vi "FFT x(t) to dB,Degrees (1D).vi"(8 "Fs (Hz)":dbl=1.0, 11 "X":dbl[](array[numeric]) format="%.2f") -> (0 "Freq (Hz)":dbl[](array[numeric]), 2 "+Freq Phase of FFT (degrees)":dbl[](array[numeric]) format="%.2f", 3 "+Freq. Mag of FFT (dB rms)":dbl[](array[numeric]) format="%.2f")   [LabVIEW 2020]
uses:
  <vilib>/Analysis/2dsp.llb/Real FFT.vi
  fea094be-e35f-4e8d-ad5d-9d99f41f383c.vi
  LinSpace (x0-dx-npts).vi
  <vilib>/Analysis/NI_AALPro.lvlib
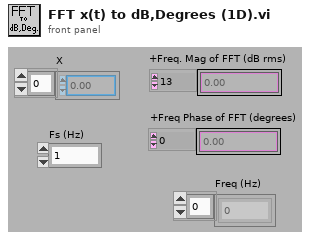
[diagram p1: front panel]
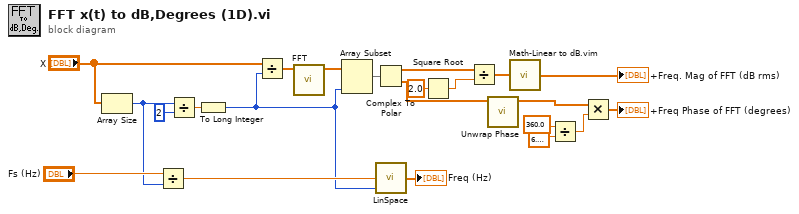
[diagram p0: block diagram]
diagram:
  n1 = Array Size(array="X") -> (size(s)=w5:i32)
  n2 = Divide(x="Fs (Hz)", y=w5) -> (x/y=w4:dbl)
  n3 = Divide(x=w5, y=2) -> (x/y=w3:dbl)
  n4 = To Long Integer(number=w3) -> (32bit integer=w1:i32)
  n5 = Divide(x="X", y=w1) -> (x/y=w9:dbl[])
  n6 = call-poly <vilib>:"FFT.vi"("X"=w9) -> ("FFT {X}"=w20:cdb[])  [unwired: 9 in, 1 out]
  n7 = Array Subset(array=w20, length=w1) -> (w21:cdb[])  [unwired: 1 in]
  n8 = Complex To Polar(r * e^(i*theta)=w21) -> (r=w15:dbl[], theta=w12:dbl[])
  n9 = call-poly "LinSpace.vi"("npts"=w1, "dx"=w4) -> ("Array"=→"Freq (Hz)":dbl[])  [unwired: 2 in, 1 out]
  n10 = Square Root(x=2.0) -> (sqrt(x)=w16:dbl)
  n11 = Divide(x=w15, y=w16) -> (x/y=w14:dbl[])
  n12 = call <vilib>:"Unwrap Phase.vi"("Phase"=w12) -> ("Unwrapped Phase"=w11:dbl[])  [unwired: 9 in, 1 out]
  n13 = call "Math-Linear to dB.vim"("linear"=w14) -> ("dB"=→"+Freq. Mag of FFT (dB rms)":dbl[])
  n14 = Divide(x=360.0, y=6.283185307179586) -> (x/y=w13:dbl)
  n15 = Multiply(x=w11, y=w13) -> (x*y=→"+Freq Phase of FFT (degrees)":dbl[])
